vi "create default alias.vi"(8 "error in":errorcluster, 11 "configuration in":refnum<class "Device Configuration.lvclass">) -> (0 "error out":errorcluster, 2 "default alias":string, 3 "configuration out":refnum<class "Device Configuration.lvclass">)   [LabVIEW 2014, in "Device Configuration.lvclass"]
uses:
  Device Configuration.lvclass
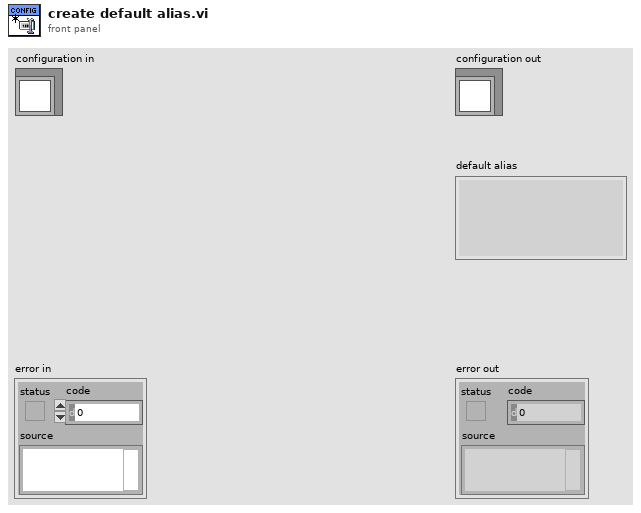
[diagram p1: front panel]
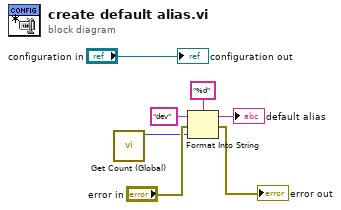
[diagram p0: block diagram]
diagram:
  n1 = call "Get Count (Global).vi"() -> ("Count"=w1:u32)  [unwired: 11 in]
  n2 = Format Into String(format string="%d", initial string="dev" ("default alias"), error in="error in", w1) -> (resulting string=→"default alias":string, error out=→"error out":errorcluster)
  "configuration out" <- "configuration in"
